vi "niRFUtil CAL Store Calibration Data.vi"(0 "Calibration Path Name":T2="dut_to_vsa", 5 "Calibration Data":T3 {"Calibration Table" min=0 max=127 format="%.2p"; "Time Stamp (sec)" format="%^.2e"; "Temperature (C)" format="%.1f"}, 11 "error in (no error)":errorcluster, 12 "Folder Path":T1) -> (15 "error out":errorcluster)   [LabVIEW 2015, in "niRFUtil.lvlib"]
doc: "This utility stores the calibration data to a file to the directory this VI is located at. The file is unique to the RF signal analyzer's serial number.\n\n(c) Copyright 2006, National Instruments, Inc. This VI may not be duplicated, sold, or distributed without written consent from National Instruments."
uses:
  niRFUtil.lvlib
  Includes/niRFUtil INC Calibration Data.ctl
  Includes/niRFUtil INC Calibration Table.ctl
  Includes/niRFUtil INC Calibration Signal Path Name.ctl
  Includes/niRFUtil INC Calibration File Path Folder.ctl
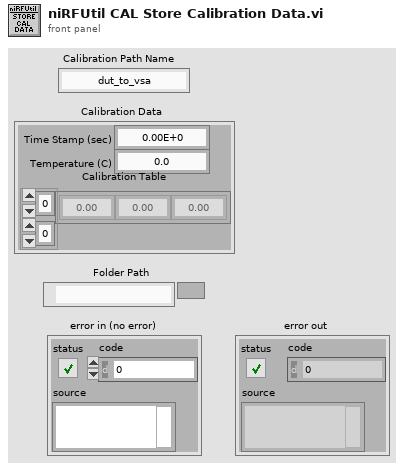
[diagram p1: front panel]
types:
  T1 = typedef "niRFUtil.lvlib/niRFUtil INC Calibration File Path Folder.ctl" = path
  T2 = typedef "niRFUtil.lvlib/niRFUtil INC Calibration Signal Path Name.ctl" = string
  T3 = typedef "niRFUtil.lvlib/niRFUtil INC Calibration Data.ctl" = cluster{"Temperature (C)":dbl, "Time Stamp (sec)":dbl, "Calibration Table":T4}
  T4 = typedef "niRFUtil.lvlib/niRFUtil INC Calibration Table.ctl" = sgl[][]
  T5 = enum16{"open", "replace", "create", "open or create", "replace or create", "replace or create with confirmation"}
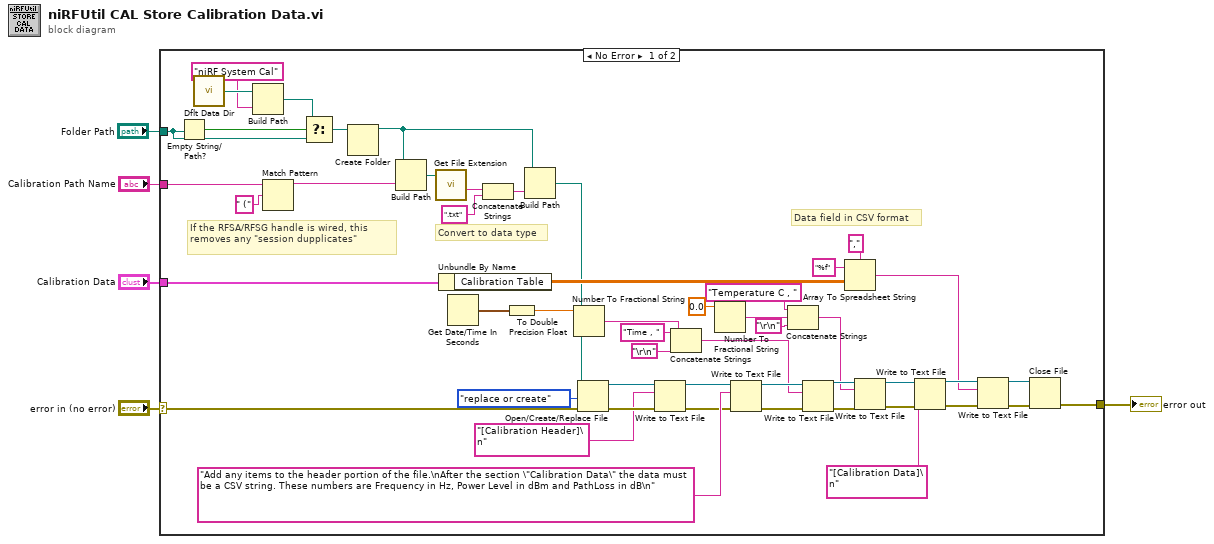
[diagram p0: block diagram]
diagram:
  n1 = case shown="No Error" "error in (no error)" {
    selector: "error in (no error)" -> [w19 w57]
    tunnel: [w17 w57] -> w4
    tunnel: "Calibration Data" -> [w16 _]
    tunnel: "Calibration Path Name" -> [w12 _]
    tunnel: "Folder Path" -> [w14 _]
    frame No Error {
      # "If the RFSA/RFSG handle is wired, this removes any \"session dupplicates\""
      # "Data field in CSV format"
      # "Convert to data type"
      n2 = Empty String/Path?(string/path=w14) -> (empty?=w15:bool)
      n3 = call <vilib>:"Dflt Data Dir.vi"() -> ("App:Default Data Directory"=w10:path)
      n4 = Build Path(base path=w10, name or relative path="niRF System Cal") -> (appended path=w8:path)
      n5 = Match Pattern(string=w12, regular expression=" (") -> (before substring=w11:T2)  [unwired: 1 in, 3 out]
      n6 = Select(t=w8, s=w15, f=w14) -> (s? t:f=w7:T1)
      n7 = Create Folder(path (use dialog)=w7) -> (created path=w6:path)  [unwired: 2 in, 2 out]
      n8 = Build Path(base path=w6, name or relative path=w11) -> (appended path=w53:path)
      n9 = call <vilib>:"Get File Extension.vi"("file"=w53) -> ("filename without extension"=w54:string)  [unwired: 1 in, 9 out]
      n10 = Unbundle By Name(w16) -> ("Calibration Table"=w28:T4)
      n11 = Get Date/Time In Seconds() -> (seconds since 1Jan1904=w52:timestamp)
      n12 = Concatenate Strings(w54, ".txt" ("string")) -> (w56:string)
      n13 = To Double Precision Float(number=w52) -> (double precision float=w27:dbl)
      n14 = Build Path(base path=w6, name or relative path=w56) -> (appended path=w20:path)
      n15 = Number To Fractional String(number=w27) -> (F-format string=w44:string)  [unwired: 3 in]
      n16 = Open/Create/Replace File(file path (use dialog)=w20, error in=w19, operation (0:open)=T5."replace or create") -> (refnum out=w25:refnum<file>, error out=w24:errorcluster)  [unwired: 3 in, 1 out]
      n17 = Write to Text File(file (use dialog)=w25, text="[Calibration Header]\n" ("delimiter (Tab)"), error in=w24) -> (refnum out=w22:refnum<file>, error out=w23:errorcluster)  [unwired: 1 in, 1 out]
      n18 = Concatenate Strings("Time , " ("string"), w44, "\r\n") -> (w30:string)
      n19 = Number To Fractional String(number=0.0) -> (F-format string=w48:string)  [unwired: 3 in]
      n20 = Write to Text File(file (use dialog)=w22, text="Add any items to the header portion of the file.\nAfter the section \"Calibration Data\" the data must be a CSV string. These numbers are Frequency in Hz, Power Level in dBm and PathLoss in dB\n" ("delimiter (Tab)"), error in=w23) -> (refnum out=w46:refnum<file>, error out=w45:errorcluster)  [unwired: 1 in, 1 out]
      n21 = Concatenate Strings("Temperature C , " ("string"), w48, "\r\n") -> (w29:string)
      n22 = Write to Text File(file (use dialog)=w46, text=w30, error in=w45) -> (refnum out=w42:refnum<file>, error out=w41:errorcluster)  [unwired: 1 in, 1 out]
      n23 = Array To Spreadsheet String(delimiter (Tab)=",", array=w28, 3:"%f" ("format string")) -> (spreadsheet string=w34:string)
      n24 = Write to Text File(file (use dialog)=w42, text=w29, error in=w41) -> (refnum out=w38:refnum<file>, error out=w37:errorcluster)  [unwired: 1 in, 1 out]
      n25 = Write to Text File(file (use dialog)=w38, text="[Calibration Data]\n" ("delimiter (Tab)"), error in=w37) -> (refnum out=w35:refnum<file>, error out=w36:errorcluster)  [unwired: 1 in, 1 out]
      n26 = Write to Text File(file (use dialog)=w35, text=w34, error in=w36) -> (refnum out=w33:refnum<file>, error out=w32:errorcluster)  [unwired: 1 in, 1 out]
      n27 = Close File(refnum=w33, error in=w32) -> (error out=w17:errorcluster)  [unwired: 1 out]
    }
    frame Error {
    }
  }
  "error out" <- w4
